vi "Listen.vi"(8 "error in (no error)":errorcluster, 11 "CIFTemplatePlugin in":refnum<class "Template_Plugin.lvclass">) -> (0 "error out":errorcluster, 3 "CIFTemplatePlugin out":refnum<class "Template_Plugin.lvclass">)   [LabVIEW 2021, in "Template_Plugin.lvclass"]
uses:
  Template_Plugin.lvclass
  Template_Plugin.lvclass/Template_Plugin.ctl
  <vilib>/CIF Foundation/CIF Core/CIFCore/Class/CIFCorePlugin.lvclass
  <vilib>/CIF Foundation/CIF Core/CIFCore/Class/Typedef/Energized States.ctl
  C:/Program Files/National Instruments/LabVIEW 2021/vi.lib/CIF Foundation/CIF Core/CIFCore/Class/CIFCorePlugin.lvclass
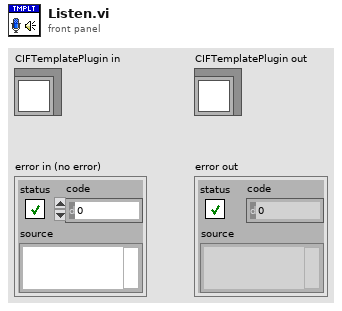
[diagram p1: front panel]
types:
  T1 = typedef "CIFCorePlugin.lvclass/Energized States.ctl" = enum16{"Listen", "Prepare", "Execute", "Housekeep", "Cleanup", "Destroy"}
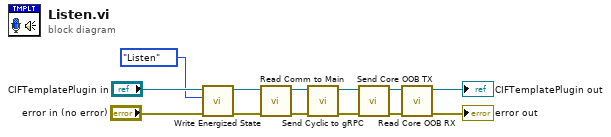
[diagram p0: block diagram]
diagram:
  n1 = call <vilib>:"Write Energized State.vi"("error in (no error)"="error in (no error)", "Energized State"=Energized_States."Listen", "CIFCorePlugin in"="CIFTemplatePlugin in") -> ("error out"=w10:errorcluster, "CIFCorePlugin out"=w11:refnum<class "Template_Plugin.lvclass">)  [unwired: 7 in]
  n2 = call "Read Comm to Main.vi"("error in (no error)"=w10, "CIFTemplatePlugin in"=w11) -> ("error out"=w2:errorcluster, "CIFTemplatePlugin out"=w1:refnum<class "Template_Plugin.lvclass">)  [unwired: 8 in]
  n3 = call "Send Cyclic to gRPC.vi"("error in (no error)"=w2, "CIFTemplatePlugin in"=w1) -> ("error out"=w6:errorcluster, "CIFTemplatePlugin out"=w7:refnum<class "Template_Plugin.lvclass">)  [unwired: 8 in]
  n4 = call <vilib>:"Send Core OOB TX.vi"("error in (no error)"=w6, "CIFCorePlugin in"=w7) -> ("error out"=w8:errorcluster, "CIFCorePlugin in"=w3:refnum<class "Template_Plugin.lvclass">)  [unwired: 8 in]
  n5 = call <vilib>:"Read Core OOB RX.vi"("error in (no error)"=w8, "CIFCorePlugin in"=w3) -> ("error out"=→"error out":errorcluster, "CIFCorePlugin in"=→"CIFTemplatePlugin out":refnum<class "Template_Plugin.lvclass">)  [unwired: 8 in]
